vi "Multiply_AI_5761_32bit_output.vi"(8 "Input Valid (T)":bool=TRUE, 9 "DDS sample":fxp<+/-,16,0>, 10 "Analog in":i16, 11 "factor":u16) -> (1 "output valid":bool, 2 "Output":fxp<+/-,32,14>)   [LabVIEW 2025]
uses:
  <vilib>/rvi/FXPMathLib/FxpConvert/subVIs/nifxpmath_Convert_SimConfig.ctl
  <vilib>/fxp/LVFixedPointQuantizationPolicyTypeDef.ctl
  <vilib>/fxp/LVFixedPointOverflowPolicyTypeDef.ctl
  <vilib>/rvi/FXPMathLib/FxpConvert/simVIs/DllFxpConvertTemp_sub.vi
  <vilib>/rvi/FXPMathLib/FxpInterpret/XNode/nifxpmath_Interpret.xnode
  <vilib>/rvi/FXPMathLib/FxpConvert/XNode/nifxpmath_Convert.xnode
  <vilib>/rvi/FXPMathLib/FxpMul/XNode/nifxpmath_Multiplier.xnode
  <vilib>/rvi/FXPMathLib/sim/FxpSim.dll
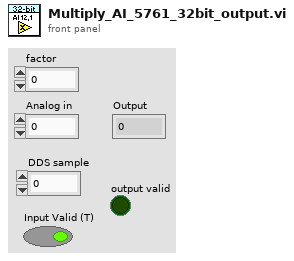
[diagram p1: front panel]
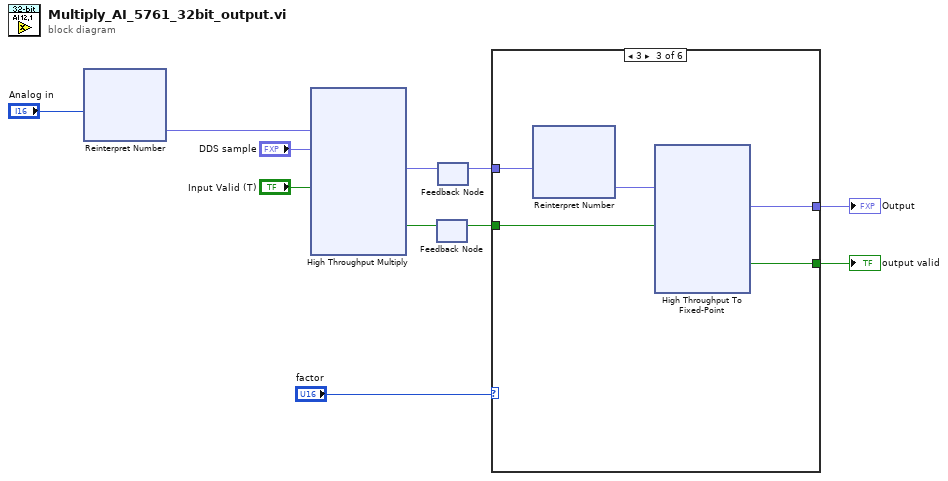
[diagram p0: block diagram]
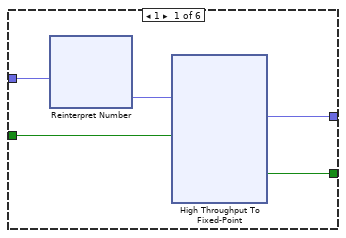
[diagram p2: hidden frame]
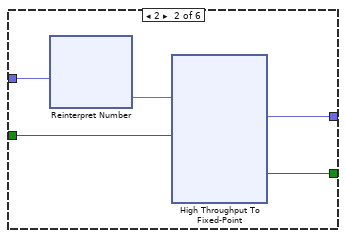
[diagram p3: hidden frame]
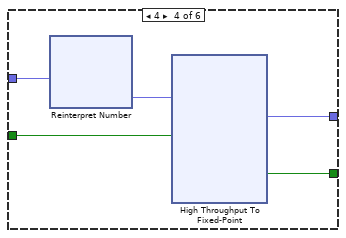
[diagram p4: hidden frame]
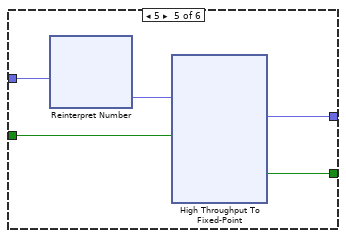
[diagram p5: hidden frame]
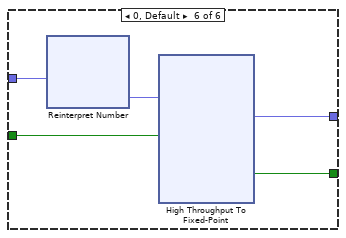
[diagram p6: hidden frame]
diagram:
  n1 = xnode "Reinterpret Number"("x"="Analog in") -> ("y"=w1:fxp<+/-,16,16>)
  n2 = xnode ("High Throughput Multiply")("x"=w1, "y"="DDS sample", "input valid"="Input Valid (T)") -> ("x*y"=w10:fxp<+/-,32,14>, "output valid"=w8:bool)  [unwired: 1 in, 1 out]
  n3 = feedback #1() -> (w6:bool)  [unwired: 1 in]
  n4 = feedback-in #1(w8) -> ()
  n5 = feedback #2() -> (w7:fxp<+/-,32,14>)  [unwired: 1 in]
  n6 = feedback-in #2(w10) -> ()
  n7 = case shown="3" "factor" {
    tunnel: w7 -> [w16 w45 w74 w103 w132 w160]
    tunnel: w6 -> [w15 w44 w73 w102 w131 w159]
    tunnel: [w14 w43 w72 w101 w130 w157] -> w5
    tunnel: [w13 w42 w71 w100 w129 w158] -> w4
    frame 1 {
      n8 = xnode "Reinterpret Number"("x"=w16) -> ("y"=w12:fxp<+/-,32,15>)
      n9 = xnode "High Throughput To Fixed-Point"("x"=w12, "input valid"=w15) -> ("y"=w13:fxp<+/-,32,14>, "output valid"=w14:bool)  [unwired: 1 in, 1 out]
    }
    frame 2 {
      n10 = xnode "Reinterpret Number"("x"=w45) -> ("y"=w41:fxp<+/-,32,16>)
      n11 = xnode "High Throughput To Fixed-Point"("x"=w41, "input valid"=w44) -> ("y"=w42:fxp<+/-,32,14>, "output valid"=w43:bool)  [unwired: 1 in, 1 out]
    }
    frame 3 {
      n12 = xnode "Reinterpret Number"("x"=w74) -> ("y"=w70:fxp<+/-,32,17>)
      n13 = xnode "High Throughput To Fixed-Point"("x"=w70, "input valid"=w73) -> ("y"=w71:fxp<+/-,32,14>, "output valid"=w72:bool)  [unwired: 1 in, 1 out]
    }
    frame 4 {
      n14 = xnode "Reinterpret Number"("x"=w103) -> ("y"=w99:fxp<+/-,32,18>)
      n15 = xnode "High Throughput To Fixed-Point"("x"=w99, "input valid"=w102) -> ("y"=w100:fxp<+/-,32,14>, "output valid"=w101:bool)  [unwired: 1 in, 1 out]
    }
    frame 5 {
      n16 = xnode "Reinterpret Number"("x"=w132) -> ("y"=w128:fxp<+/-,32,19>)
      n17 = xnode "High Throughput To Fixed-Point"("x"=w128, "input valid"=w131) -> ("y"=w129:fxp<+/-,32,14>, "output valid"=w130:bool)  [unwired: 1 in, 1 out]
    }
    frame 0, Default {
      n18 = xnode "Reinterpret Number"("x"=w160) -> ("y"=w161:fxp<+/-,32,14>)
      n19 = xnode "High Throughput To Fixed-Point"("x"=w161, "input valid"=w159) -> ("y"=w158:fxp<+/-,32,14>, "output valid"=w157:bool)  [unwired: 1 in, 1 out]
    }
  }
  "Output" <- w4
  "output valid" <- w5
